vi "newFinal.vi"(8 "error in (no error)":errorcluster, 11 "MagSpec_Bella in":refnum<class "MagSpec_Bella.lvclass">) -> (0 "error out":errorcluster, 3 "MagSpec_Bella out":refnum<class "MagSpec_Bella.lvclass">)   [LabVIEW 2020, in "MagSpec_Bella.lvclass"]
uses:
  MagSpec_Bella.lvclass
  MagSpec_Bella.lvclass/MagSpec_Bella.ctl
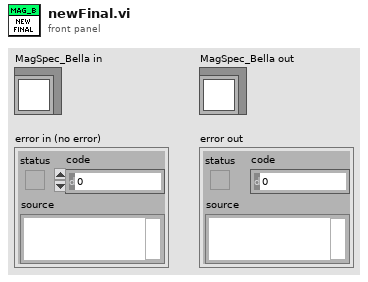
[diagram p1: front panel]
types:
  T1 = typedef "finalCalib--Cluster.ctl" = cluster{"X":dbl[][], "xi":dbl[][], "delta momentum":dbl, "Y":dbl[][], "yi":dbl[][], "angle (Y)":dbl[], "delta angle":dbl, "scale delta angle":dbl, "intraX":dbl, "intraY":dbl, "mask":dbl[][]}
  T2 = typedef "Calibration_Pixel_based.ctl" = cluster{"y1(pixel)":dbl[], "y2(pixel)":dbl[], "dp/B [MeV/C/B] (pixel)":dbl[], "energyDependence Input(pixel)":dbl[], "bending angle [deg](pixel)":dbl[], "total path(pixel)":dbl[], "pixel angle (y)(pixel)":dbl[], "energy dependence (pixel)":dbl[], "charge compensation (pixel)":dbl[], "Momentum [MeV/C](pixel)":dbl[], "angular compensation(pixel)":dbl[]}
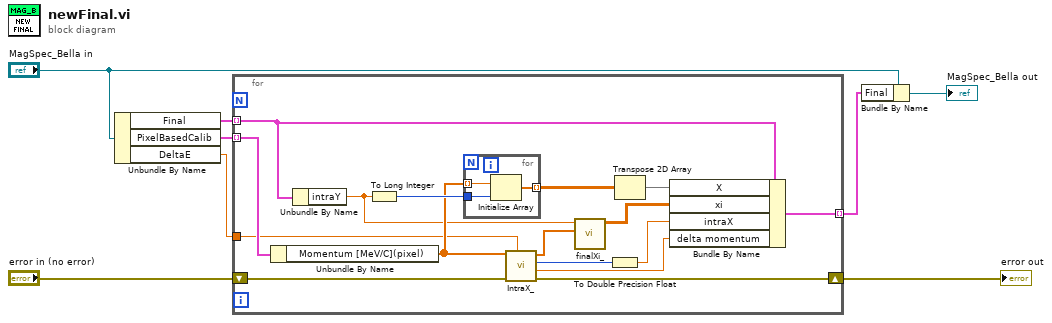
[diagram p0: block diagram]
diagram:
  n1 = Unbundle By Name("MagSpec_Bella in") -> ("Final"=w5:T1[], "PixelBasedCalib"=w2:T2[], "DeltaE"=w1:dbl)
  n2 = for {
    shift-right: [w18] -> w4
    shift-left: "error in (no error)" -> [w23]
    tunnel: w2 -> [w17] mode=indexing
    tunnel: w5 -> [w15] mode=indexing
    tunnel: [w14] -> w7 mode=indexing
    tunnel: w1 -> [w9]
    n3 = Unbundle By Name(w17) -> ("Momentum [MeV/C](pixel)"=w16:dbl[])
    n4 = Unbundle By Name(w15) -> ("intraY"=w12:dbl)
    n5 = To Long Integer(number=w12) -> (32bit integer=w21:i32)
    n6 = for {
      tunnel: w16 -> [w27] mode=indexing
      tunnel: w21 -> [w26]
      tunnel: [w25] -> w20 mode=indexing
      n7 = Initialize Array(w27, w26) -> (w25:dbl[])
    }
    n8 = call "IntraX_.vi"("DeltaE"=w9, "error in (no error)"=w23, "Momentum [MeV/C](pixel)"=w16) -> ("error out"=w18:errorcluster, "delta momentum"=w13:dbl, "IntraX"=w11:i32, "Ramp Pattern"=w22:dbl[])  [unwired: 5 in]
    n9 = call "finalXi_.vi"("Ramp Pattern"=w22, "intraY"=w12) -> ("Array"=w24:dbl[][])  [unwired: 9 in]
    n10 = To Double Precision Float(number=w11) -> (double precision float=w10:dbl)
    n11 = Transpose 2D Array(2D array=w20) -> (transposed array=w19:dbl[][])
    n12 = Bundle By Name(cluster=w15, "X"=w19, "xi"=w24, "intraX"=w10, "delta momentum"=w13) -> (w14:T1)
  }
  "error out" <- w4
  n13 = Bundle By Name(cluster="MagSpec_Bella in", "Final"=w7) -> (→"MagSpec_Bella out":refnum<class "MagSpec_Bella.lvclass">)
